vi "AIDI-Create Tasks (DI).vi"(0 "DI":T1, 5 "DI Device Name":tag, 7 "Sync Device Name":tag, 11 "error in":errorcluster) -> (4 "task out":refnum<k21>, 15 "error out":errorcluster)   [LabVIEW 2020]
uses:
  Typedefs/DI-Output Spec.ctl
  <vilib>/DAQmx/create/channels.llb/DAQmx Create Channel (DI-Digital Input).vi
  <vilib>/DAQmx/configure/timing.llb/DAQmx Timing (Sample Clock).vi
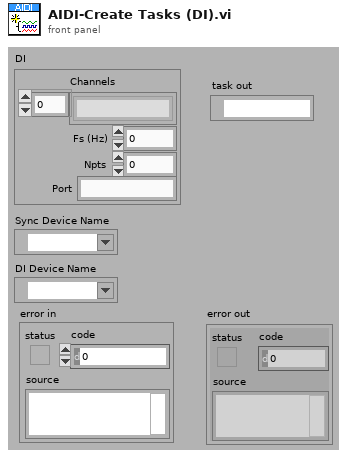
[diagram p1: front panel]
types:
  T1 = typedef "DI-Output Spec.ctl" = cluster{"Channels":string[], "Fs (Hz)":dbl, "Npts":i32, "Port":string}
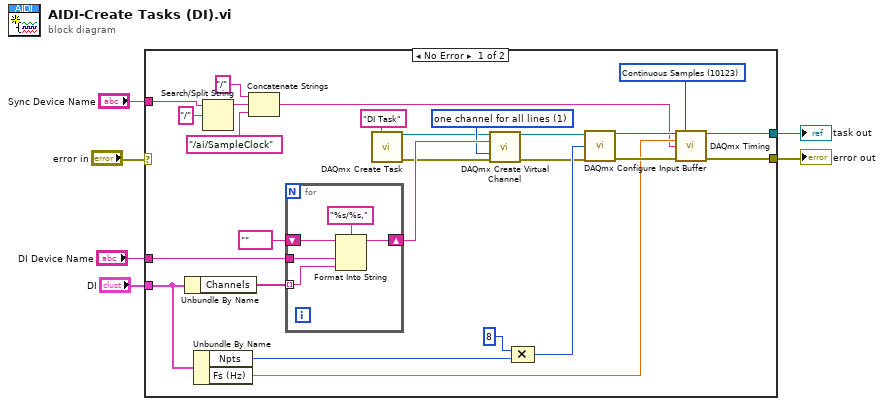
[diagram p0: block diagram]
diagram:
  n1 = case shown="No Error" "error in" {
    selector: "error in" -> [_ w38]
    tunnel: "DI Device Name" -> [w14 _]
    tunnel: [w25 w38] -> w4
    tunnel: "DI" -> [w19 _]
    tunnel: [w16 _] -> w2
    tunnel: "Sync Device Name" -> [w8 _]
    frame No Error {
      w23 = 1 items=["one channel for each line", "one channel for all lines"] ("line grouping")
      w28 = 10123 items=["Finite Samples"=10178, "Continuous Samples"=10123, "Hardware Timed Single Point"=12522] ("sample mode")
      n2 = Unbundle By Name(w19) -> ("Channels"=w30:string[])
      n3 = Unbundle By Name(w19) -> ("Npts"=w17:i32, "Fs (Hz)"=w18:dbl)
      n4 = Search/Split String(string=w8, search string/char (-)="/") -> (substring before match=w13:string)  [unwired: 1 in, 2 out]
      n5 = Concatenate Strings("/", w13, "/ai/SampleClock") -> (w7:string)
      n6 = for {
        tunnel: w30 -> [w33] mode=indexing
        shift-right: [w35] -> w27
        shift-left: tag "" ("DAQmx Physical Channel") -> [w36]
        tunnel: w14 -> [w34]
        n7 = Format Into String(format string="%s/%s,", initial string=w36, w34, w33) -> (resulting string=w35:string)  [unwired: 1 in, 1 out]
      }
      n8 = call <vilib>:"DAQmx Create Task.vi"("new task name"="DI Task" ("name to assign")) -> ("task out"=w10:refnum<k21>, "error out"=w9:errorcluster)  [unwired: 13 in]
      n9 = call-poly <vilib>:"DAQmx Create Virtual Channel.vi"("task in"=w10, "lines"=w27, "line grouping"=w23, "error in"=w9) -> ("task out"=w22:refnum<k21>, "error out"=w21:errorcluster)  [unwired: 10 in]
      n10 = Compound Arithmetic op=MULTIPLY(8 ("x"), w17) -> (w24:i32)
      n11 = call <vilib>:"DAQmx Configure Input Buffer.vi"("task/channels in"=w22, "buffer size (in samples per channel)"=w24, "error in"=w21) -> ("task out"=w15:refnum<k21>, "error out"=w20:errorcluster)  [unwired: 11 in]
      n12 = call-poly <vilib>:"DAQmx Timing.vi"("task/channels in"=w15, "sample mode"=w28, "rate"=w18, "source"=w7, "error in"=w20) -> ("task out"=w16:refnum<k21>, "error out"=w25:errorcluster)  [unwired: 9 in]
    }
    frame Error {
    }
  }
  "error out" <- w4
  "task out" <- w2
